vi "Deposit.vi"(8 "error in (no error)":errorcluster, 10 "Amount":dbl, 11 "AChecking in":refnum<class "AChecking.lvclass">) -> (0 "error out":errorcluster, 2 "Balance":dbl, 3 "AChecking out":refnum<class "AChecking.lvclass">)   [LabVIEW 2020, in "AChecking.lvclass"]
uses:
  AChecking.lvclass
  AChecking.lvclass/AChecking.ctl
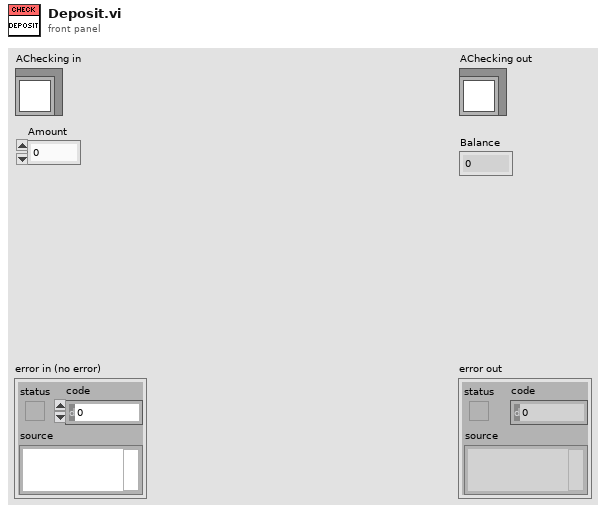
[diagram p1: front panel]
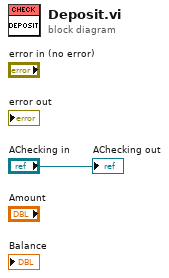
[diagram p0: block diagram]
diagram:
  "AChecking out" <- "AChecking in"
